vi "Test.vi"() -> ()   [LabVIEW 2020]
uses:
  Test program data.ctl
  Lock-in-amplifier/Libraries/Lock-in amplifier/Lock-in amplifier.lvlib
  Monochromator/Libraries/Monochromator/Monochromator.lvlib
panel:
  out "XY Graph":cluster{"X":dbl, "Y":dbl}[](graph)
  out "Data":dbl caption="Dato leído"
  out "Current position":dbl caption="Posición actual"
  in  "Connect":bool
  in  "Move":bool
  in  "Set speed":bool
  in  "Velocidad":dbl=100.0 format="%#_g nm/min"
  in  "Posición":dbl=400.0 format="%#_g nm"
  in  "stop":bool
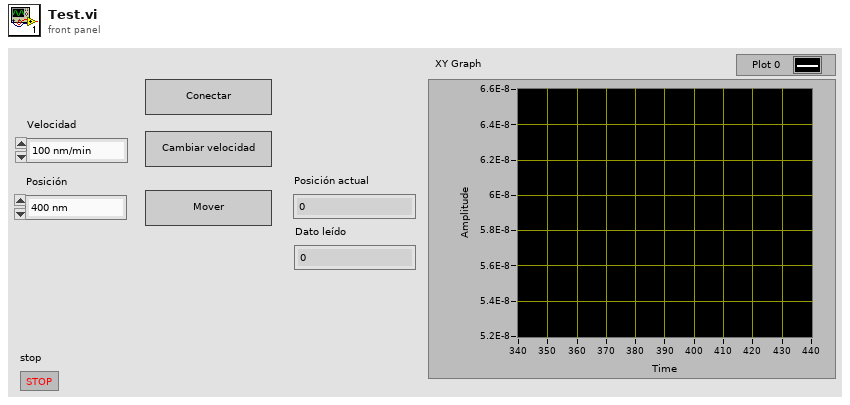
[diagram p1: front panel]
types:
  T1 = typedef "Test program data.ctl" = cluster{"Lock-in ID":i32, "Mono ID":i32}
  T2 = typedef "Lock-in amplifier.lvlib/Broadcast Events--cluster.ctl" = cluster{"Module Did Init":refnum<user-event>, "Status Updated":refnum<user-event>, "Error Reported":refnum<user-event>, "Module Did Stop":refnum<user-event>, "Update Module Execution Status":refnum<user-event>, "Helper Loop Status Updated":refnum<user-event>}
  T3 = typedef "Monochromator.lvlib/Broadcast Events--cluster.ctl" = cluster{"Module Did Init":refnum<user-event>, "Status Updated":refnum<user-event>, "Error Reported":refnum<user-event>, "Module Did Stop":refnum<user-event>, "Update Module Execution Status":refnum<user-event>, "Helper Loop Status Updated":refnum<user-event>, "Data read":refnum<user-event>}
  T4 = cluster{"baud rate":u32, "data bits":u16, "parity":enum16{"None", "Odd", "Even", "Mark", "Space"}, "stop bits":u16}
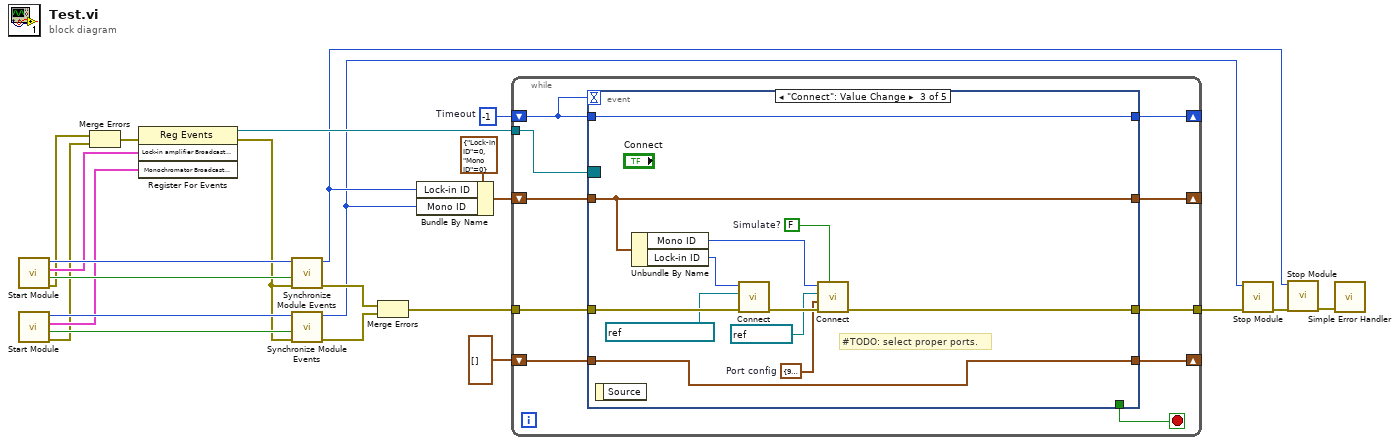
[diagram p0: block diagram]
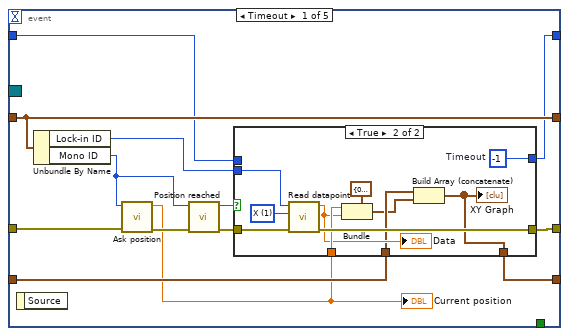
[diagram p2: hidden frame]
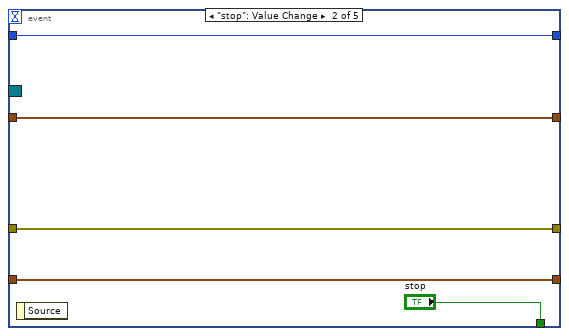
[diagram p4: hidden frame]
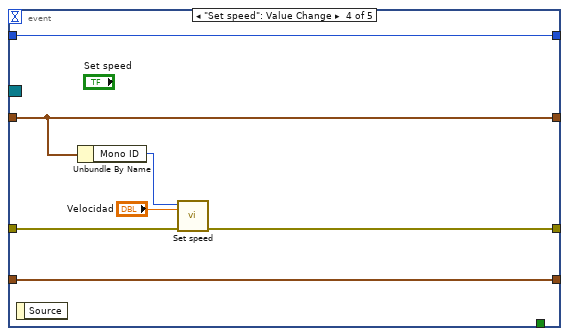
[diagram p5: hidden frame]
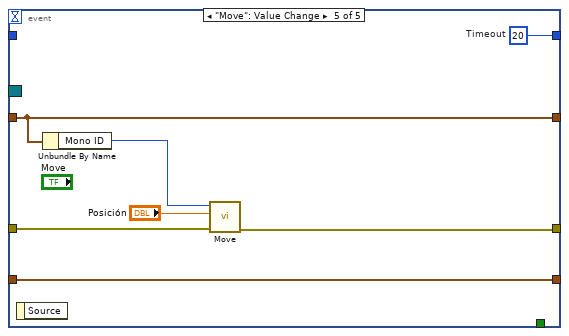
[diagram p6: hidden frame]
diagram:
  w2 = -1  # Timeout
  n1 = call "Start Module.vi"() -> ("error out"=w13:errorcluster, "Wait for Event Sync?"=w22:bool, "Lock-in amplifier Broadcast Events"=w16:T2, "Module ID"=w23:i32)  [unwired: 8 in]
  n2 = call "Start Module.vi"() -> ("error out"=w12:errorcluster, "Wait for Event Sync?"=w20:bool, "Monochromator Broadcast Events"=w15:T3, "Module ID"=w21:i32)  [unwired: 8 in]
  n3 = Merge Errors(w13, w12) -> (w14:errorcluster)
  n4 = register-events(error in=w14, w16, w15) -> (reference out=w10:refnum<event-registration>, error out=w11:errorcluster)  [unwired: 1 in]
  n5 = call "Synchronize Module Events.vi"("error in"=w11, "Wait for Event Sync?"=w22, "Module ID in"=w23) -> ("error out"=w19:errorcluster, "Module ID out"=w5:i32)  [unwired: 7 in]
  n6 = call "Synchronize Module Events.vi"("error in"=w11, "Wait for Event Sync?"=w20, "Module ID in"=w21) -> ("error out"=w18:errorcluster, "Module ID out"=w4:i32)  [unwired: 7 in]
  n7 = Merge Errors(w19, w18) -> (w17:errorcluster)
  n8 = Bundle By Name(cluster=T1 {"Lock-in ID"=0, "Mono ID"=0}, "Lock-in ID"=w5, "Mono ID"=w4) -> (w3:T1)
  n9 = while {
    tunnel: w17 -> [w32]
    tunnel: [w31] -> w9
    tunnel: w10 -> [w30]
    shift-right: [w28] -> _
    shift-left: w3 -> [w29]
    shift-right: [w26] -> _
    shift-left: w2 -> [w27]
    shift-right: [w24] -> _
    shift-left: cluster{"X":dbl, "Y":dbl}[] [] ("XY Graph") -> [w25]
    stop <- w33 stop-if-true
    n10 = event shown="[2] \"Connect\": Value Change" {
      selector: w30 -> [_ _ _ _ _]
      dyn-events: _ -> [_ _ _ _ _]
      timeout: w27 -> [_ _ _ _ _]
      tunnel: [_ "stop" _ _ _] -> w33
      tunnel: w32 -> [w45 w64 w76 w84 w91]
      tunnel: [w41 w64 w68 w83 w90] -> w31
      tunnel: w29 -> [w46 w63 w77 w81 w89]
      tunnel: [w46 w63 w77 w81 w89] -> w28
      tunnel: w27 -> [w38 w62 w67 w79 _]
      tunnel: [w37 w62 w67 w79 w86] -> w26
      tunnel: w25 -> [w36 w61 w66 w78 w85]
      tunnel: [w34 w61 w66 w78 w85] -> w24
      event Timeout {
        n11 = event-data() -> ()  [unwired: 1 in, 1 out]
        n12 = Unbundle By Name(w46) -> ("Lock-in ID"=w39:i32, "Mono ID"=w43:i32)
        n13 = call "Ask position.vi"("error in"=w45, "Module ID"=w43) -> ("error out"=w44:errorcluster, "Current position"=w35:dbl)  [unwired: 7 in, 1 out]
        "Current position" <- w35
        n14 = call "Position reached.vi"("error in"=w44, "Module ID"=w43) -> ("error out"=w42:errorcluster, "Done?"=w40:bool)  [unwired: 7 in, 1 out]
        n15 = case shown="True" w40 {
          tunnel: w42 -> [w49 w60]
          tunnel: [w49 w59] -> w41
          tunnel: w39 -> [_ w58]
          tunnel: w38 -> [w48 _]
          tunnel: [w48 w56] -> w37
          tunnel: w36 -> [w47 w52]
          tunnel: w35 -> [_ w54]
          tunnel: [w47 w50] -> w34
          frame False {
          }
          frame True {
            w56 = -1  # Timeout
            w57 = u16 1 items=["X"=1, "Y"=2, "R"=3, "Theta"=4, "Channel 1"=5, "Channel 2"=6, "Aux In 1"=7, "Aux In 2"=8, "Aux In 3"=9, "Aux In 4"=10] ("Parameter")
            n16 = call "Read datapoint.vi"("error in"=w60, "Parameter"=w57, "Module ID"=w58) -> ("error out"=w59:errorcluster, "Data"=w53:dbl)  [unwired: 6 in, 1 out]
            "Data" <- w53
            n17 = Bundle(cluster=cluster{"X":dbl, "Y":dbl} {"X"=0.0, "Y"=0.0}, "X"=w54, "Y"=w53) -> (w51:cluster{"X":dbl, "Y":dbl})
            n18 = Build Array (concatenate)(w52, w51) -> (w50:cluster{"X":dbl, "Y":dbl}[])
            "XY Graph" <- w50
          }
        }
      }
      event "stop": Value Change {
        n19 = event-data() -> ()  [unwired: 1 in, 1 out]
      }
      event "Connect": Value Change {
        w71 = FALSE  # Simulate?
        w72 = T4 {"baud rate"=9600, "data bits"=8, "parity"=enum."None", "stop bits"=10}  # Port config
        # "#TODO: select proper ports."
        n20 = event-data() -> ()  [unwired: 1 in, 1 out]
        n21 = Unbundle By Name(w77) -> ("Mono ID"=w73:i32, "Lock-in ID"=w74:i32)
        n22 = call "Connect.vi"("error in"=w76, "VISA resource name"=refnum<visa-resource-name> "GPIB0::8::INSTR", "Module ID"=w74) -> ("error out"=w75:errorcluster)  [unwired: 6 in, 2 out]
        n23 = call "Connect.vi"("Simulate?"=w71, "error in"=w75, "Port config"=w72, "VISA resource name"=refnum<visa-resource-name> "COM7", "Module ID"=w73) -> ("error out"=w68:errorcluster)  [unwired: 4 in, 2 out]
      }
      event "Set speed": Value Change {
        n24 = event-data() -> ()  [unwired: 1 in, 1 out]
        n25 = Unbundle By Name(w81) -> ("Mono ID"=w80:i32)
        n26 = call "Set speed.vi"("error in"=w84, "nm/min"="Velocidad", "Module ID"=w80) -> ("error out"=w83:errorcluster)  [unwired: 8 in]
      }
      event "Move": Value Change {
        w86 = 20  # Timeout
        n27 = event-data() -> ()  [unwired: 1 in, 1 out]
        n28 = Unbundle By Name(w89) -> ("Mono ID"=w88:i32)
        n29 = call "Move.vi"("error in"=w91, "Wavelength"="Posición", "Module ID"=w88) -> ("error out"=w90:errorcluster)  [unwired: 8 in]
      }
    }
  }
  n30 = call "Stop Module.vi"("error in"=w9, "Module ID"=w4) -> ("error out"=w8:errorcluster)  [unwired: 9 in]
  n31 = call "Stop Module.vi"("error in"=w8, "Module ID"=w5) -> ("error out"=w7:errorcluster)  [unwired: 9 in]
  n32 = call <vilib>:"Simple Error Handler.vi"("error in (no error)"=w7) -> ()  [unwired: 4 in, 5 out]
